vi "write_text.vi"() -> ()   [LabVIEW 2019]
panel:
  in  "Start":bool
  out "error out":errorcluster
  in  "text":string
  in  "file path":path
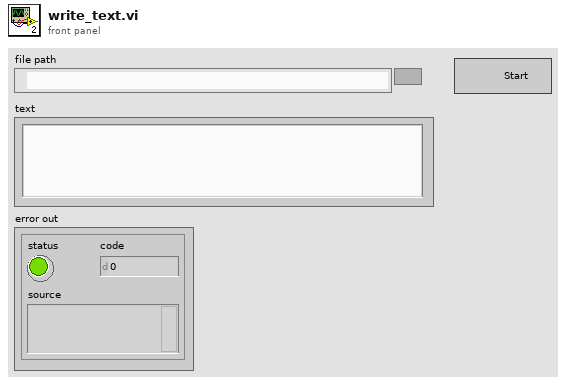
[diagram p1: front panel]
types:
  T1 = enum16{"open", "replace", "create", "open or create", "replace or create", "replace or create with confirmation"}
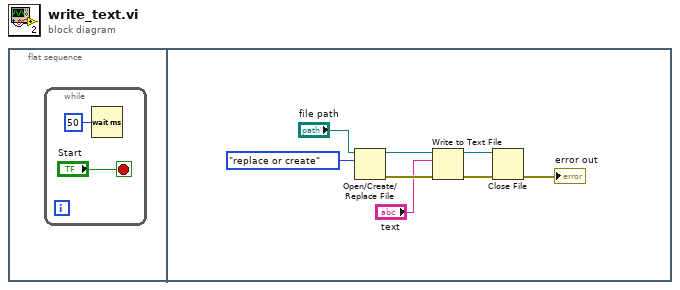
[diagram p0: block diagram]
diagram:
  n1 = flat-sequence {
    frame #0 {
      n2 = while {
        stop <- "Start" stop-if-true
        n3 = Wait (ms)(milliseconds to wait=u32 50) -> ()  [unwired: 1 out]
      }
    }
    frame #1 {
      n4 = Open/Create/Replace File(file path (use dialog)="file path", operation (0:open)=T1."replace or create") -> (refnum out=w8:refnum<file>, error out=w7:errorcluster)  [unwired: 4 in, 1 out]
      n5 = Write to Text File(file (use dialog)=w8, text="text", error in=w7) -> (refnum out=w6:refnum<file>, error out=w5:errorcluster)  [unwired: 1 in, 1 out]
      n6 = Close File(refnum=w6, error in=w5) -> (error out=→"error out":errorcluster)  [unwired: 1 out]
    }
  }
